vi "FEA_Model_Pinned_BC.vi"(10 "Pin Location":i32, 11 "FEA_Model in":refnum<class "FEA_Model.lvclass">) -> (2 "K Matrix":dbl[][](array[numeric]), 3 "M Matrix":dbl[][](array[numeric]))   [LabVIEW 2021, in "FEA_Model.lvclass"]
uses:
  FEA_Model.lvclass
  FEA_Model.lvclass/FEA_Model.ctl
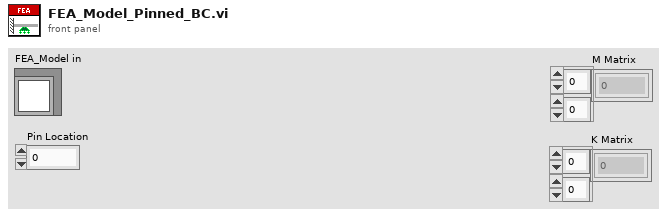
[diagram p1: front panel]
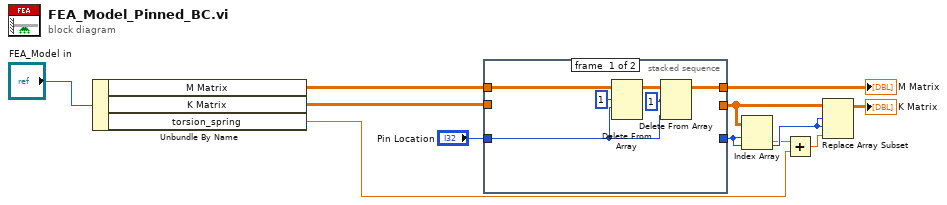
[diagram p0: block diagram]
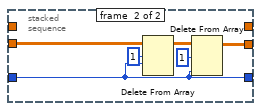
[diagram p2: hidden frame]
diagram:
  n1 = Unbundle By Name("FEA_Model in") -> ("M Matrix"=w10:dbl[][], "K Matrix"=w9:dbl[][], "torsion_spring"=w6:dbl)
  n2 = stacked-sequence {
    tunnel: [w17 _] -> w3
    tunnel: w10 -> [w14 _]
    tunnel: "Pin Location" -> [w12 w18]
    tunnel: w9 -> [_ w20]
    tunnel: [_ w19] -> w8
    tunnel: [_ w18] -> w7
    frame #0 {
      n3 = Delete From Array(array=w14, length=1, index (row)=w12) -> (array with subset deleted=w16:dbl[][])  [unwired: 1 in, 1 out]
      n4 = Delete From Array(array=w16, length=1, index (col)=w12) -> (array with subset deleted=w17:dbl[][])  [unwired: 1 in, 1 out]
    }
    frame #1 {
      n5 = Delete From Array(array=w20, length=1, index (row)=w18) -> (array with subset deleted=w23:dbl[][])  [unwired: 1 in, 1 out]
      n6 = Delete From Array(array=w23, length=1, index (col)=w18) -> (array with subset deleted=w19:dbl[][])  [unwired: 1 in, 1 out]
    }
  }
  "M Matrix" <- w3
  n7 = Index Array(array=w8, index (row)=w7, index (col)=w7) -> (element=w5:dbl)
  n8 = Add(x=w5, y=w6) -> (x+y=w4:dbl)
  n9 = Replace Array Subset(array=w8, new element=w4, index (row)=w7, index (col)=w7) -> (→"K Matrix":dbl[][])
